vi "pointer.condition.normal.vi"(7 "Pointer methods":T1, 8 "error in (no error)":errorcluster, 11 "TestCase in":refnum<class "TestCase.Pointer.lvclass">) -> (0 "error out":errorcluster, 3 "TestCase out":refnum<class "TestCase.Pointer.lvclass">)   [LabVIEW 2016, in "TestCase.Pointer.lvclass"]
uses:
  TestCase.Pointer.lvclass
  pointer methods.ctl
  TestCase.Pointer.lvclass/TestCase.Pointer.ctl
  Source/Classes/Pointer/Memory.Pointer.lvclass
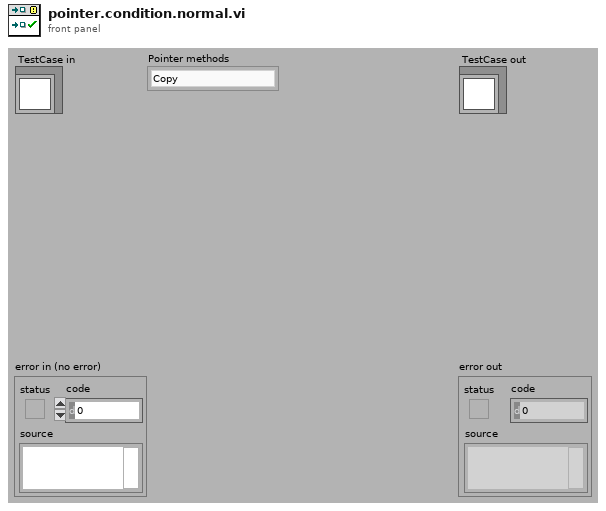
[diagram p1: front panel]
types:
  T1 = typedef "TestCase.Pointer.lvclass/pointer methods.ctl" = enum16{"Copy"}
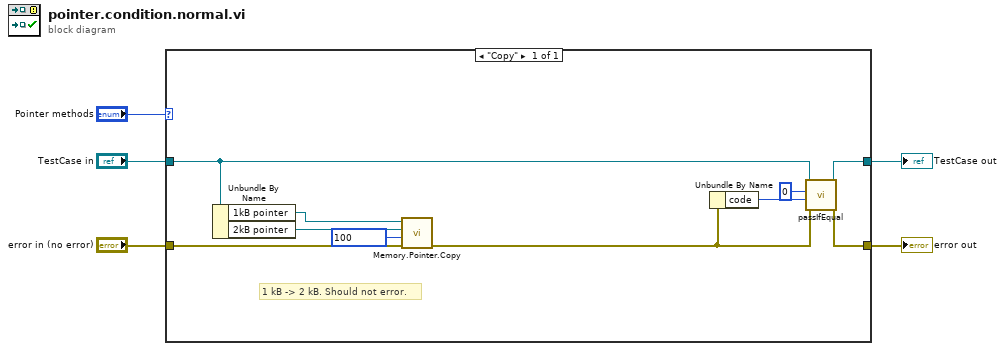
[diagram p0: block diagram]
diagram:
  n1 = case shown="\"Copy\"" "Pointer methods" {
    tunnel: "error in (no error)" -> [w11]
    tunnel: [w15] -> w4
    tunnel: "TestCase in" -> [w6]
    tunnel: [w14] -> w2
    frame "Copy" {
      # "1 kB -> 2 kB. Should not error."
      n2 = Unbundle By Name(w6) -> ("1kB pointer"=w9:refnum<class "Memory.Pointer.lvclass">, "2kB pointer"=w8:refnum<class "Memory.Pointer.lvclass">)
      n3 = call "Memory.Pointer.Copy.vi"("error in (no error)"=w11, "bytes to copy"=u64 100, "dst Pointer in"=w8, "src Pointer in"=w9) -> ("error out"=w10:errorcluster)  [unwired: 4 in, 3 out]
      n4 = Unbundle By Name(w10) -> ("code"=w13:i32)
      n5 = call-dynamic "passIfEqual.vi"("error in (no error)"=w10, "y"=w13, "x"=0 ("code"), "TestCase in"=w6) -> ("error out"=w15:errorcluster, "TestCase out"=w14:refnum<class "TestCase.Pointer.lvclass">)  [unwired: 6 in]
    }
  }
  "error out" <- w4
  "TestCase out" <- w2
